vi "FormatStrings.vi"() -> ()   [LabVIEW 2019]
panel:
  out "error out":errorcluster
  out "Graph":dbl[](graph)
  in  "Provide your desired string":string
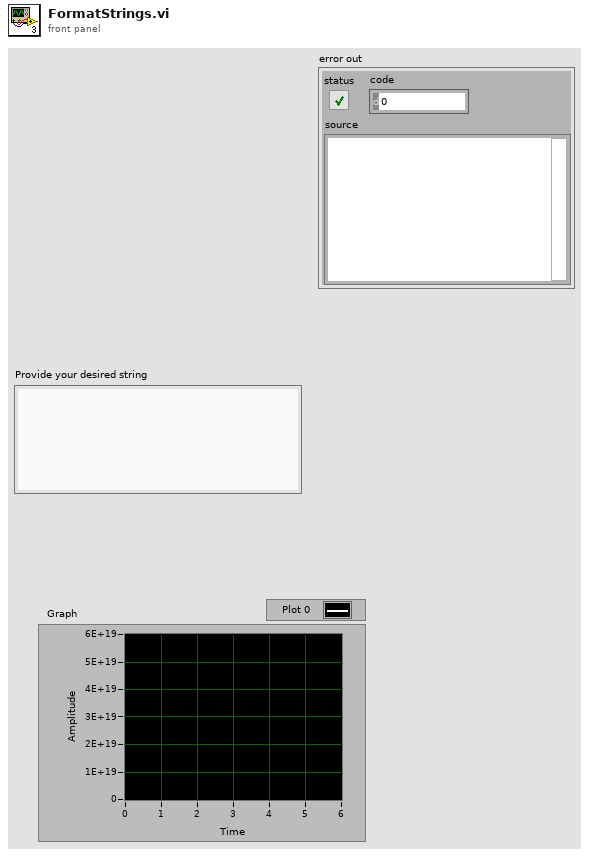
[diagram p1: front panel]
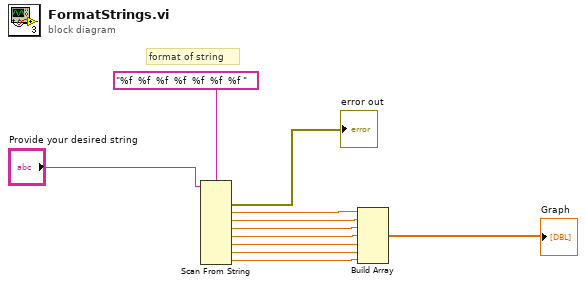
[diagram p0: block diagram]
diagram:
  # "format of string"
  n1 = Scan From String(format string="%f  %f  %f  %f  %f  %f  %f ", input string="Provide your desired string") -> (error out=→"error out":errorcluster, output 1=w9:dbl, output 2=w8:dbl, output 3=w7:dbl, output 4=w6:dbl, output 5=w5:dbl, output 6=w4:dbl, output 7=w3:dbl)  [unwired: 9 in, 2 out]
  n2 = Build Array(w9, w8, w7, w6, w5, w4, w3) -> (→"Graph":dbl[])
